vi "onLock.vi"(8 "error in (no error)":errorcluster, 10 "Player In":refnum<class "Player.lvclass">, 11 "PlayingState in":refnum<class "PlayingState.lvclass">) -> (0 "error out":errorcluster, 1 "String":string, 2 "Player Out":refnum<class "Player.lvclass">, 3 "PlayingState out":refnum<class "PlayingState.lvclass">)   [LabVIEW 2018, in "PlayingState.lvclass"]
uses:
  PlayingState.lvclass
  Player Class/Player.lvclass
  LockedState Class/LockedState.lvclass
  C:/Users/fflores/Documents/LabVIEW-Open-Projects/LabIVEW OOP Design Patterns/State Pattern/State Class/State.lvclass
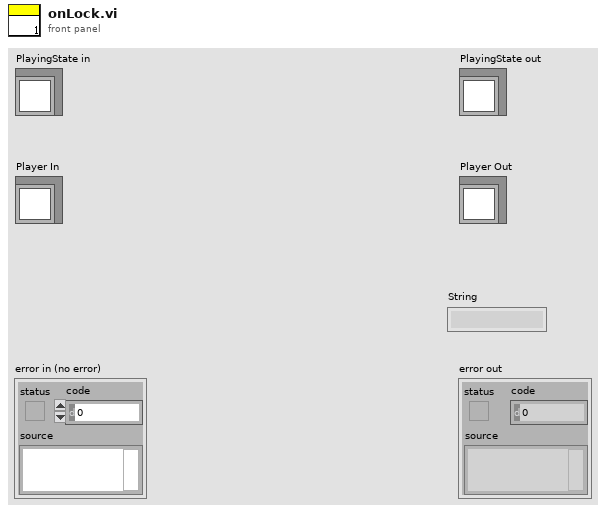
[diagram p1: front panel]
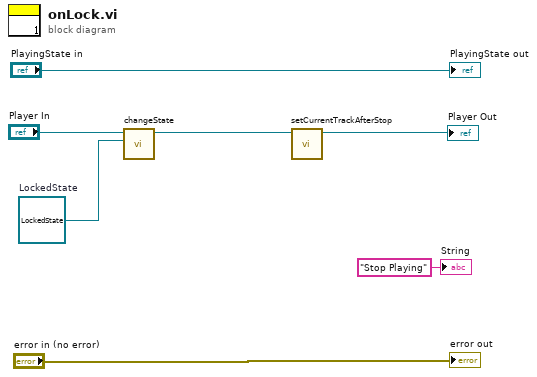
[diagram p0: block diagram]
diagram:
  w3 = refnum<class "LockedState.lvclass"> refnum  # LockedState
  n1 = call-dynamic "changeState.vi"("State"=w3, "Player in"="Player In") -> ("Player out"=w4:refnum<class "Player.lvclass">)  [unwired: 8 in, 1 out]
  n2 = call-dynamic "setCurrentTrackAfterStop.vi"("Player in"=w4) -> ("Player out"=→"Player Out":refnum<class "Player.lvclass">)  [unwired: 9 in, 1 out]
  "error out" <- "error in (no error)"
  "PlayingState out" <- "PlayingState in"
  "String" <- "Stop Playing" ("String")
